vi "RSZVB Read To File From Instrument.vi"(8 "error in (no error)":errorcluster {"code" format="%.0x"}, 9 "Destination (\\test.hcp)":path=path "C:/test.hcp", 10 "Source (D:\\user\\data\\test.hcp)":path=path "D:/user/data/test.hcp", 11 "VISA session":refnum<visa-resource-name>) -> (0 "error out":errorcluster {"code" format="%.0x"}, 3 "dup VISA session":refnum<visa-resource-name>)   [LabVIEW 2011]
doc: "This VI is used to read data from the instrument and write it to a user specified file on the host computer.\n\nRemote-control command(s):\nMMEMory:DATA? '<file_name>'"
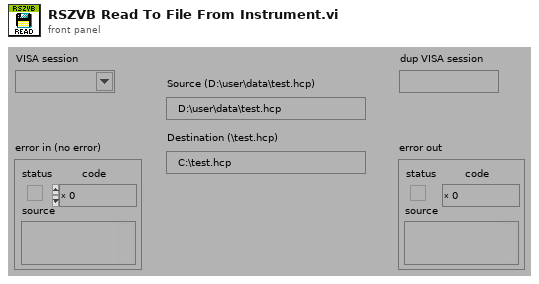
[diagram p1: front panel]
types:
  T1 = enum16{"open", "replace", "create", "open or create", "replace or create", "replace or create with confirmation"}
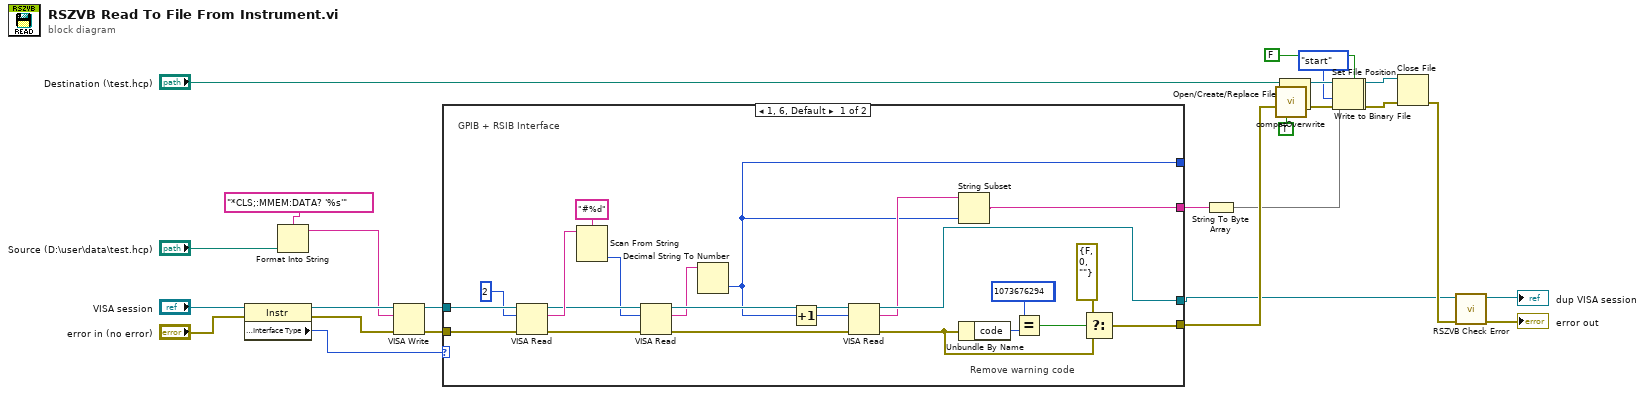
[diagram p0: block diagram]
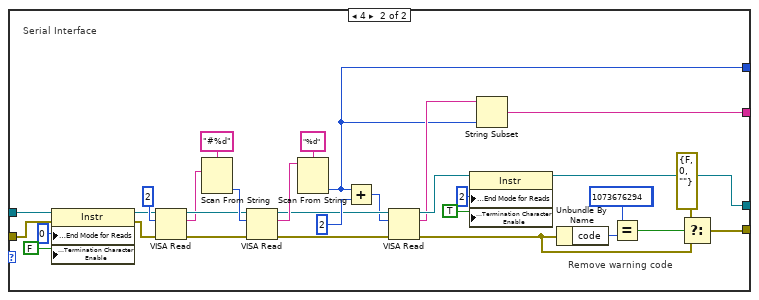
[diagram p2: hidden frame]
diagram:
  n1 = property class="Instr"(reference="VISA session", error in="error in (no error)") -> (reference out=w23:refnum<visa-resource-name>, error out=w24:errorcluster, "Interface Information:Interface Type"=w28:u16)
  n2 = Format Into String(format string="*CLS;:MMEM:DATA? '%s'", "Source (D:\\user\\data\\test.hcp)") -> (resulting string=w18:string)  [unwired: 2 in, 1 out]
  n3 = VISA Write(VISA resource name=w23, write buffer=w18, error in (no error)=w24) -> (VISA resource name out=w22:refnum<visa-resource-name>, error out=w21:errorcluster)  [unwired: 1 out]
  n4 = case shown="1, 6, Default" w28 {
    tunnel: w21 -> [w50 w68]
    tunnel: w22 -> [w49 w69]
    tunnel: [w29 w57] -> _
    tunnel: [w39 w54] -> w13
    tunnel: [w31 w59] -> w25
    tunnel: [w34 w60] -> w7
    frame 1, 6, Default {
      (unwired) 1073676294
      # "Remove warning code"
      # "GPIB + RSIB Interface"
      n5 = VISA Read(VISA resource name=w49, byte count=u32 2 ("byte count (0)"), error in (no error)=w50) -> (VISA resource name out=w45:refnum<visa-resource-name>, read buffer=w48:string, error out=w44:errorcluster)  [unwired: 1 out]
      n6 = Scan From String(format string="#%d", input string=w48) -> (output 1=w35:i32)  [unwired: 3 in, 3 out]
      n7 = VISA Read(VISA resource name=w45, byte count=w35, error in (no error)=w44) -> (VISA resource name out=w38:refnum<visa-resource-name>, read buffer=w36:string, error out=w37:errorcluster)  [unwired: 1 out]
      n8 = Decimal String To Number(string=w36) -> (number=w29:i32)  [unwired: 2 in, 1 out]
      n9 = Increment(x=w29) -> (x+1=w32:i32)
      n10 = VISA Read(VISA resource name=w38, byte count=w32, error in (no error)=w37) -> (VISA resource name out=w34:refnum<visa-resource-name>, read buffer=w30:string, error out=w33:errorcluster)  [unwired: 1 out]
      n11 = String Subset(string=w30, length (rest)=w29) -> (substring=w31:string)  [unwired: 1 in]
      n12 = Unbundle By Name(w33) -> ("code"=w43:i32)
      n13 = Equal?(x=1073676294, y=w43) -> (x = y?=w41:bool)
      n14 = Select(t=errorcluster {"status"=FALSE, "code"=0, "source"=""} ("error out"), s=w41, f=w33) -> (s? t:f=w39:errorcluster)
    }
    frame 4 {
      (unwired) 1073676294
      # "Remove warning code"
      # "Serial Interface"
      n15 = property class="Instr"(reference=w69, error in=w68, "Serial Settings:End Mode for Reads"=u16 0 ("ASRL End In"), "Message Based Settings:Termination Character Enable"=FALSE ("TermChar En")) -> (reference out=w72:refnum<visa-resource-name>, error out=w73:errorcluster)
      n16 = VISA Read(VISA resource name=w72, byte count=u32 2 ("byte count (0)"), error in (no error)=w73) -> (VISA resource name out=w77:refnum<visa-resource-name>, read buffer=w76:string, error out=w78:errorcluster)  [unwired: 1 out]
      n17 = Scan From String(format string="#%d", input string=w76) -> (output 1=w79:i32)  [unwired: 3 in, 3 out]
      n18 = VISA Read(VISA resource name=w77, byte count=w79, error in (no error)=w78) -> (VISA resource name out=w65:refnum<visa-resource-name>, read buffer=w80:string, error out=w66:errorcluster)  [unwired: 1 out]
      n19 = Scan From String(format string="%d", input string=w80) -> (output 1=w57:i32)  [unwired: 3 in, 3 out]
      n20 = Add(x=w57, y=2) -> (x+y=w64:i32)
      n21 = VISA Read(VISA resource name=w65, byte count=w64, error in (no error)=w66) -> (VISA resource name out=w61:refnum<visa-resource-name>, read buffer=w58:string, error out=w51:errorcluster)  [unwired: 1 out]
      n22 = property class="Instr"(reference=w61, "Serial Settings:End Mode for Reads"=u16 2 ("ASRL End In"), "Message Based Settings:Termination Character Enable"=TRUE ("TermChar En")) -> (reference out=w60:refnum<visa-resource-name>)  [unwired: 1 in, 1 out]
      n23 = String Subset(string=w58, length (rest)=w57) -> (substring=w59:string)  [unwired: 1 in]
      n24 = Unbundle By Name(w51) -> ("code"=w56:i32)
      n25 = Equal?(x=1073676294, y=w56) -> (x = y?=w53:bool)
      n26 = Select(t=errorcluster {"status"=FALSE, "code"=0, "source"=""} ("error out"), s=w53, f=w51) -> (s? t:f=w54:errorcluster)
    }
  }
  n27 = String To Byte Array(string=w25) -> (unsigned byte array=w11:u8[])
  n28 = call <vilib>:"compatOverwrite.vi"("overwrite (F)"=TRUE) -> ("overwrite?"=w1:T1)
  n29 = Open/Create/Replace File(file path (use dialog)="Destination (\\test.hcp)", error in=w13, operation (0:open)=w1) -> (refnum out=w17:refnum<file>, error out=w14:errorcluster)  [unwired: 3 in, 1 out]
  n30 = Set File Position(refnum=w17, from (0:start)=enum16{"start", "end", "current"}."start" ("pos mode (0:2)"), error in=w14) -> (refnum out=w4:refnum<file>, error out=w3:errorcluster)  [unwired: 1 in]
  n31 = Write to Binary File(file (use dialog)=w4, data=w11, error in=w3, 5:FALSE ("prepend array or string size? (T)")) -> (refnum out=w16:refnum<file>, error out=w15:errorcluster)  [unwired: 2 in, 1 out]
  n32 = Close File(refnum=w16, error in=w15) -> (error out=w8:errorcluster)  [unwired: 1 out]
  n33 = call "RSZVB Check Error.vi"("error in (no error)"=w8, "VISA session"=w7) -> ("error out"=→"error out":errorcluster, "dup VISA session"=→"dup VISA session":refnum<visa-resource-name>)  [unwired: 8 in]
